vi "Fridge_Valve_alarm.vi"(3 "enabled":bool=TRUE, 5 "level_lo":dbl=65.0 format="%.1f", 7 "level_hi":dbl=85.0 format="%.1f", 8 "time_last_alarm_in":timestamp, 10 "readout_status":bool=TRUE, 11 "level":dbl) -> (0 "time_last_alarm_out":timestamp, 2 "alarm_status":u32(colorbox))   [LabVIEW 2019]
panel:
  out "message":string
  in  "interval":dbl=600.0
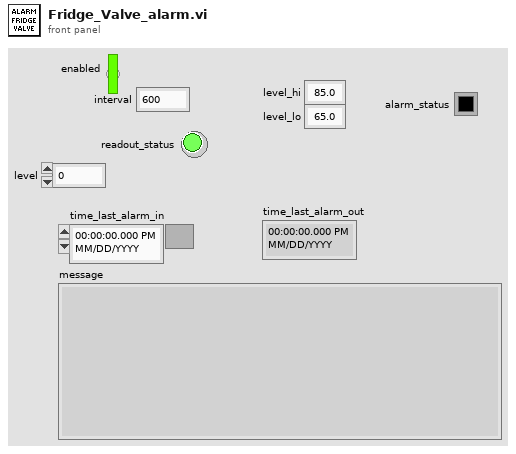
[diagram p1: front panel]
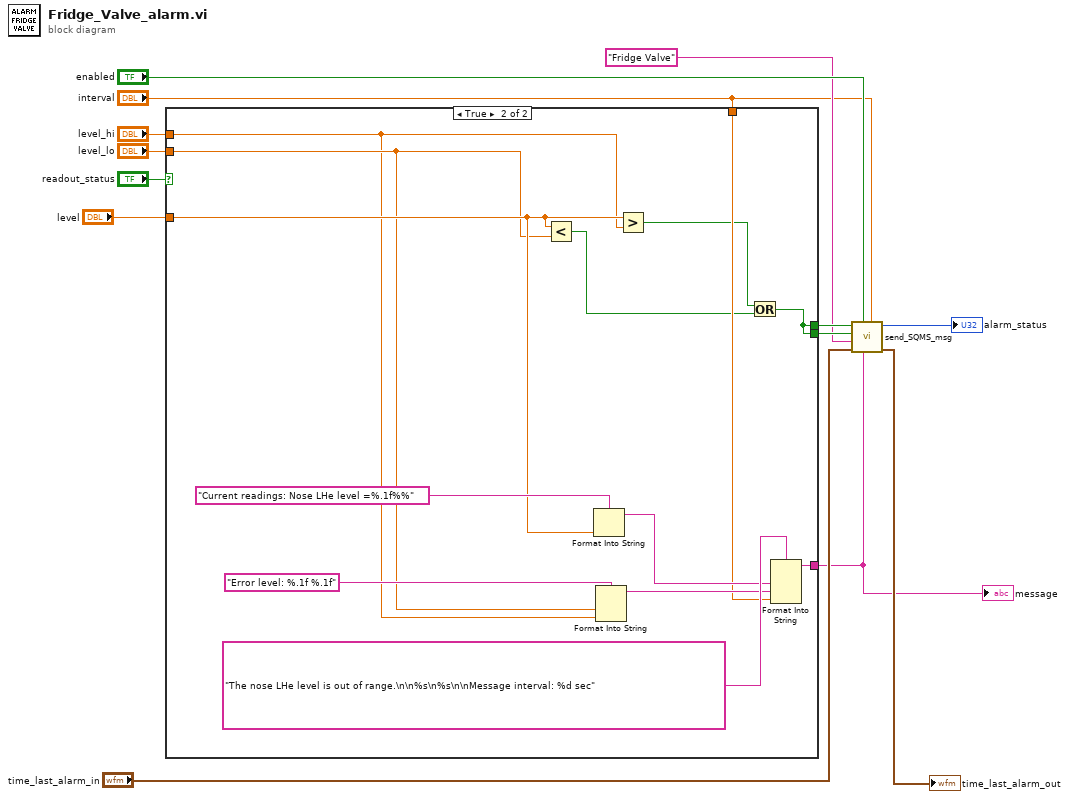
[diagram p0: block diagram]
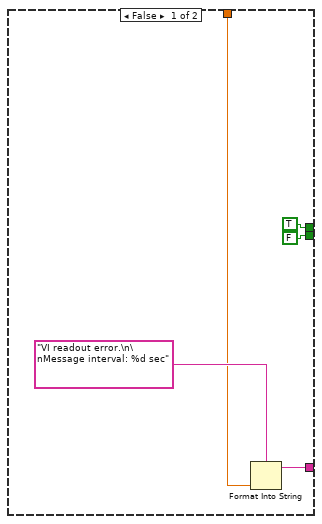
[diagram p2: hidden frame]
diagram:
  n1 = case shown="True" "readout_status" {
    tunnel: [TRUE w23] -> w12
    tunnel: [FALSE w23] -> w11
    tunnel: "level_hi" -> [_ w19]
    tunnel: "level_lo" -> [_ w20]
    tunnel: "interval" -> [w14 w26]
    tunnel: [w15 w25] -> w4
    tunnel: "level" -> [_ w24]
    frame False {
      n2 = Format Into String(format string="VI readout error.\n\nMessage interval: %d sec" ("msg"), w14) -> (resulting string=w15:string)  [unwired: 2 in, 1 out]
    }
    frame True {
      n3 = Less?(x=w24, y=w20) -> (x < y?=w21:bool)
      n4 = Format Into String(format string="Current readings: Nose LHe level =%.1f%%" ("msg"), w24) -> (resulting string=w28:string)  [unwired: 2 in, 1 out]
      n5 = Format Into String(format string="Error level: %.1f %.1f" ("msg"), w20, w19) -> (resulting string=w27:string)  [unwired: 2 in, 1 out]
      n6 = Greater?(x=w24, y=w19) -> (0:w22:bool)
      n7 = Or(x=w22, y=w21) -> (x .or. y?=w23:bool)
      n8 = Format Into String(format string="The nose LHe level is out of range.\n\n%s\n%s\n\nMessage interval: %d sec" ("msg"), w28, w27, w26) -> (resulting string=w25:string)  [unwired: 2 in, 1 out]
    }
  }
  "message" <- w4
  n9 = call "send_SQMS_msg.vi"("alarm_interval"="interval", "msg"=w4, "enabled"="enabled", "time_last_alarm_in"="time_last_alarm_in", "title"="Fridge Valve", "warning"=w11, "error"=w12) -> ("time_last_alarm_out"=→"time_last_alarm_out":timestamp, "alarm_status"=→"alarm_status":u32)  [unwired: 2 in, 1 out]
